vi "pid_plant_example.vi"() -> ()   [LabVIEW 2015]
doc: "This example shows you a classical feedback control loop with a PID controller and a simulated process that behaves as a second order transfer function. You can ignore the settings for the simulated process if you want and focus on tunning the controller. You can also change the parameters of the simulated process in order to make them behave differently (i.e. oscillate more, have less overshoot, etc)."
uses:
  <userlib>/_OpenG.lib/comparison/comparison.llb/Boolean Changed__ogtk.vi
  discrete_control_systems/discrete_control_systems.lvlib
panel:
  in  "Simulation Parameters":T1={"Gain"=2.0, "NaturalFreq (wn in Hz)"=7.0, "DampingRatio (zeta)"=0.2} caption="Second Order Simulation Parameters"
  in  "PID Parameters":cluster{"Kc":dbl, "Ti":dbl, "Td":dbl}={"Kc"=0.07, "Ti"=0.005, "Td"=0.1}
  in  "Sampling Time(s)":dbl=0.01 format="%#_13g"
  in  "Closed Loop?":enum32{"Closed Loop", "Open Loop"}(radio)
  in  "Manual Input (Open Loop)":dbl=1.0
  out "Process Chart":T2(graph)={"Set Point"=4.0, "Plant Input\n(Open Loop)"=2.000000000001828, "y(k)"=4.000000000050655}
  in  "Stop":bool
  out "Process Variable":dbl=4.000000000050655
  in  "Reset Plant":bool
  in  "Simulation Output Limits":cluster{"Max":dbl, "Min":dbl}={"Max"=200.0, "Min"=-200.0}
  out "Control Value":dbl=2.000000000001828
  in  "Set Point":dbl=2.0
  in  "PID Output Limits":cluster{"Max":dbl, "Min":dbl}={"Max"=10.0, "Min"=-10.0}
  in  "Reset Controller":bool
  # "JKI DISCRETE CONTROL SYSTEMS\nPID control example of a simulated 2nd order process\nThis example shows you a classical feedback control loop with a PID controller and a simulated process that behaves \nas a second order transfer function. You can ignore the settings for the simulated process if you want and focus on\ntunning the controller. You can also change the parameters of the simulated process in order to make them behave\ndifferently (i.e. oscillate more, have less overshoot, etc)"
  # "This is how fast is your control\nloop running. This number is used\nunder the hood for all the control\nand simulation calculations. You\ncan modify it to see how the behavior\nof the loop changes."
  # "SIMULATED PROCESS"
  # "PID CONTROLLER"
  # "You can configure the behavior of\nthe simulated process by changing\nthe parameters. This will obviously \naffect the control and may require\nretuning of the PID"
  # "You can change the setpoint\nwhen running closed loop"
  # "The manual input value goes\ndirectly to the process when running\nopen loop"
  # "Select between Closed Loop (PID is ON)\nor Open Loop (PID is OFF)"
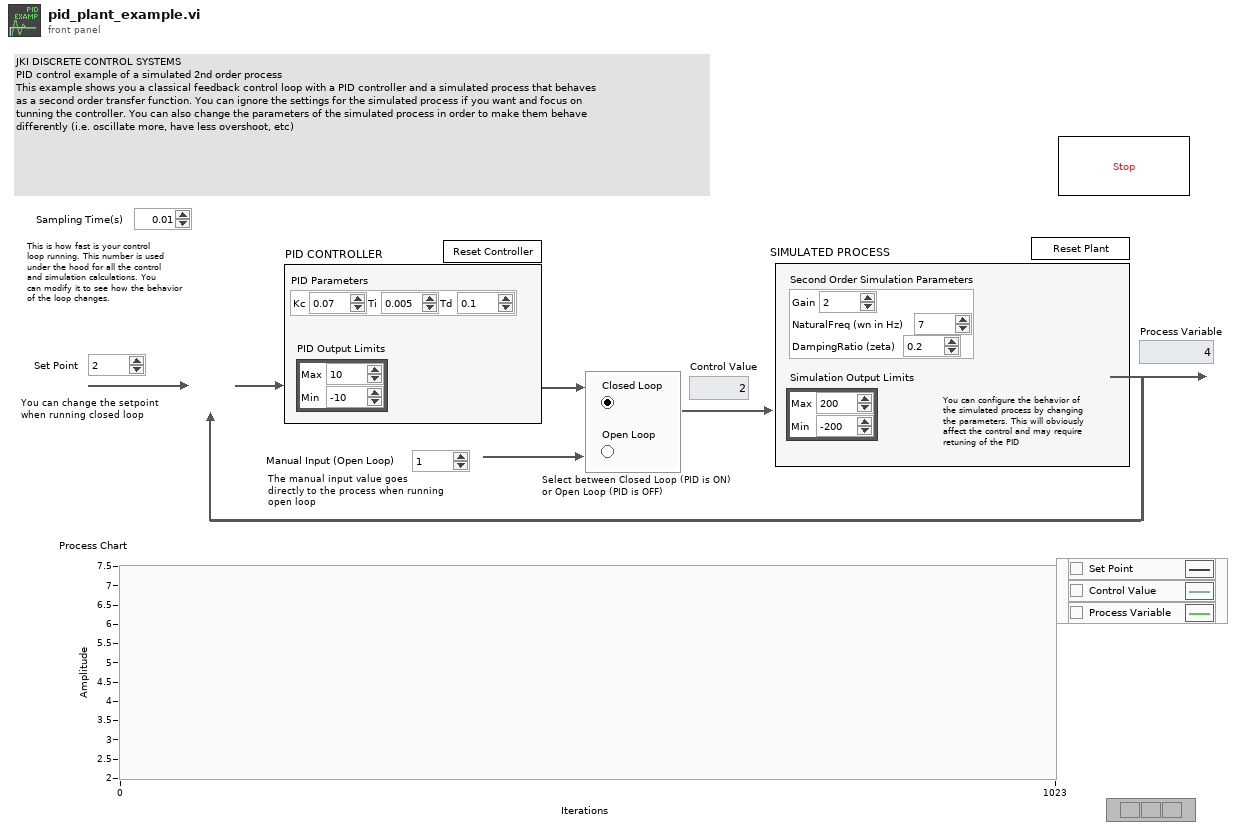
[diagram p1: front panel]
types:
  T1 = cluster{"Gain":dbl, "NaturalFreq (wn in Hz)":dbl, "DampingRatio (zeta)":dbl}
  T2 = cluster{"Set Point":dbl, "Plant Input\n(Open Loop)":dbl, "y(k)":dbl}
  T3 = cluster{"Set Point":dbl, "Manual Input (Open Loop)":dbl, "output":dbl}
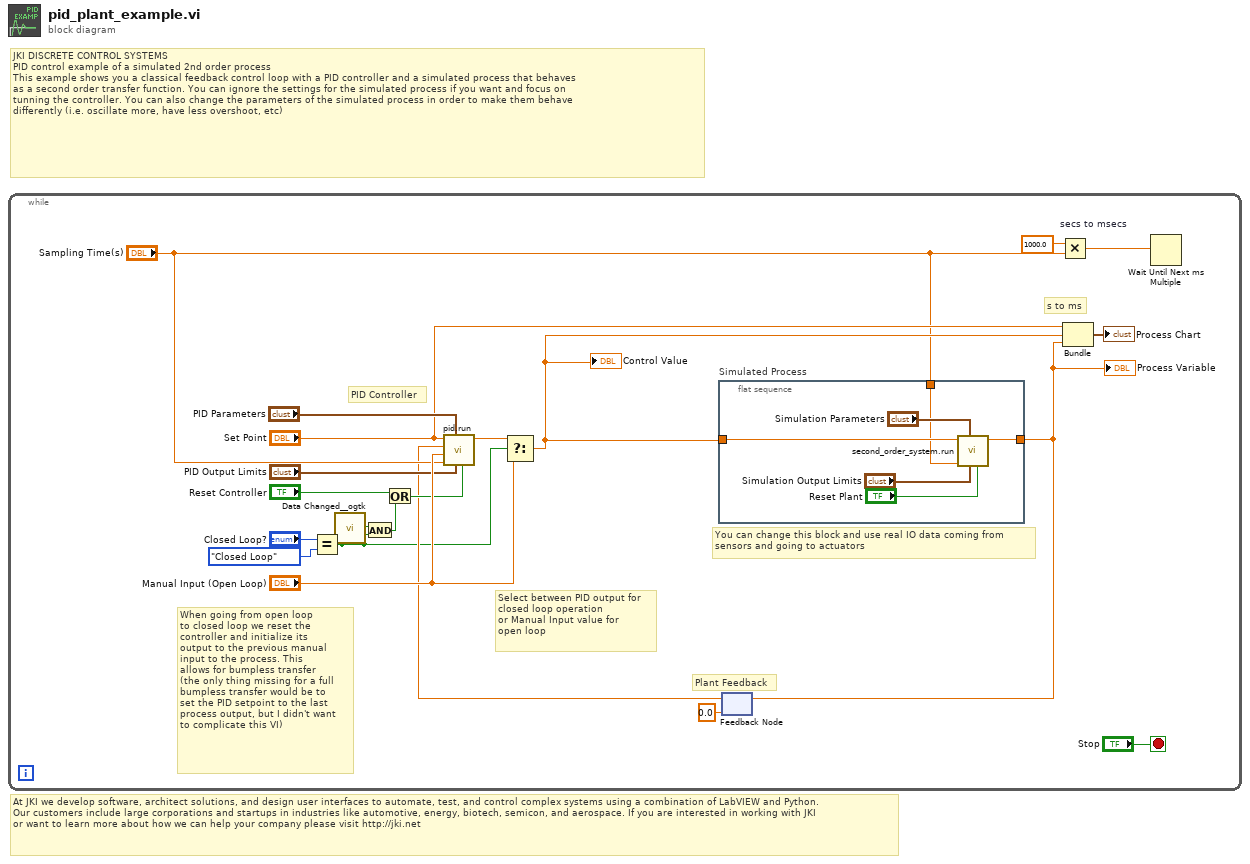
[diagram p0: block diagram]
diagram:
  # "JKI DISCRETE CONTROL SYSTEMS\nPID control example of a simulated 2nd order process\nThis example shows you a classical feedback control loop with a PID controller and a simulated process that behaves \nas a second order transfer function. You can ignore the settings for the simulated process if you want and focus on\ntunning the controller. You can also change the parameters of the simulated process in order to make them behave\ndifferently (i.e. oscillate more, have less overshoot, etc)"
  # "At JKI we develop software, architect solutions, and design user interfaces to automate, test, and control complex systems using a combination of LabVIEW and Python. \nOur customers include large corporations and startups in industries like automotive, energy, biotech, semicon, and aerospace. If you are interested in working with JKI\nor want to learn more about how we can help your company please visit http://jki.net"
  n1 = while {
    stop <- "Stop" stop-if-true
    # "PID Controller"
    # "When going from open loop\nto closed loop we reset the \ncontroller and initialize its \noutput to the previous manual\ninput to the process. This\nallows for bumpless transfer\n(the only thing missing for a full \nbumpless transfer would be to\nset the PID setpoint to the last\nprocess output, but I didn't want\nto complicate this VI)"
    # "Select between PID output for\nclosed loop operation\nor Manual Input value for \nopen loop"
    # "You can change this block and use real IO data coming from\nsensors and going to actuators"
    # "s to ms"
    # "Plant Feedback"
    n2 = Equal?(x="Closed Loop?", y=enum32{"Closed Loop", "Open Loop"}."Closed Loop") -> (x = y?=w2:bool)
    n3 = call-poly <userlib>:"Data Changed__ogtk.vi"("Boolean"=w2) -> ("Changed"=w3:bool)
    n4 = And(x=w3, y=w2) -> (x .and. y?=w1:bool)
    n5 = Or(x="Reset Controller", y=w1) -> (x .or. y?=w9:bool)
    n6 = flat-sequence "Simulated Process" {
      tunnel: w7 -> [w25]
      tunnel: [w24] -> w6
      tunnel: "Sampling Time(s)" -> [w22]
      frame #0 {
        n7 = call "second_order_system.run.vi"("reset? (F)"="Reset Plant", "output_limits (100/0)"="Simulation Output Limits", "transfer_function_parameters"="Simulation Parameters", "sampling_time (s)"=w22, "input"=w25) -> ("output"=w24:dbl)  [unwired: 6 in]
      }
    }
    n8 = feedback-in #1(w6) -> ()
    n9 = feedback #1(0.0 ("y(k)")) -> (w4:dbl)
    n10 = call "pid.run.vi"("reset? (F)"=w9, "output_limits (100/0)"="PID Output Limits", "pid_parameters"="PID Parameters", "sampling_time (s)"="Sampling Time(s)", "initial_output (0)"="Manual Input (Open Loop)", "feedback"=w4, "setpoint"="Set Point") -> ("controller_output"=w8:dbl)  [unwired: 4 in]
    n11 = Select(t=w8, s=w2, f="Manual Input (Open Loop)") -> (s? t:f=w7:dbl)
    "Control Value" <- w7
    n12 = Multiply "secs to msecs"(x=1000.0, y="Sampling Time(s)") -> (x*y=w15:dbl)
    n13 = Bundle("Set Point"="Set Point", "Manual Input (Open Loop)"=w7, "output"=w6) -> (→"Process Chart":T3)  [unwired: 1 in]
    n14 = Wait Until Next ms Multiple(millisecond multiple=w15) -> ()  [unwired: 1 out]
    "Process Variable" <- w6
  }
